vi "Discrete Lead Compensator Design.vi"() -> ()   [LabVIEW 2018]
uses:
  <vilib>/addons/Control Design/_Model Construction/Data Typedefs.llb/CD CtoD Conversion Method.ctl
  <vilib>/addons/Control Design/_Model Construction/Model Typedefs.llb/CD Transfer Function Model (MIMO).ctl
  <vilib>/addons/Control Design/_Model Construction/Model Typedefs.llb/CD General Elements.ctl
  <vilib>/addons/Control Design/_Model Construction/Model Typedefs.llb/CD Transfer Function Model (SISO).ctl
  <vilib>/addons/Control Design/_Utility/Rendering.llb/Rendering Transfer Function Options.ctl
  <vilib>/addons/Control Design/_Model Conversions/Continuous and Discrete.llb/Continuous and Discrete SubVI/cd_Convert Continuous to Discrete (TF).vi
  <vilib>/addons/Control Design/_Utility/Model Viewer.llb/Model Viewer SubVI/cd_Draw Transfer Function Equation (TF).vi
  <vilib>/addons/Control Design/_Model Construction/Model Creation.llb/Model Creation SubVI/cd_Create Transfer Function Model.vi
  <vilib>/addons/Control Design/_Model Interconnection/Model Interconnection.llb/Model Interconnection SubVI/cd_Matrix Multiply Models (TF and TF).vi
  <vilib>/addons/Control Design/_Dynamic Analysis/Dynamic Analysis.llb/Dynamic Analysis subVI/cd_Root Locus (Transfer Function).vi
  <vilib>/addons/Control Design/_Frequency Response Analysis/Frequency Response.llb/Frequency Response subVI/cd_Gain and Phase Margin (Transfer Function).vi
  <vilib>/addons/Control Design/_Model Interconnection/Model Interconnection.llb/Model Interconnection SubVI/cd_Unit Feedback (TF and TF).vi
  <vilib>/addons/Control Design/_Time Response Analysis/Time Response.llb/Time Response subVI/cd_Step Response (Transfer Function).vi
  <vilib>/addons/Control Design/_Utility/NI_CD_Model Viewer.lvlib
  <vilib>/addons/Control Design/_Model Construction/NI_LinSys_Model Typedefs.lvlib
  <vilib>/addons/Control Design/_Model Construction/NI_LinSys_Data Typedefs.lvlib
  <vilib>/addons/Control Design/_Utility/NI_LinSys_Rendering.lvlib
  <vilib>/addons/Control Design/_Model Conversions/NI_CD_Continuous and Discrete.lvlib
  <vilib>/addons/Control Design/_Dynamic Analysis/NI_CD_Dynamic Analysis.lvlib
  <vilib>/addons/Control Design/_Model Construction/NI_LinSys_Model Creation.lvlib
  <vilib>/addons/Control Design/_Model Interconnection/NI_CD_Model Interconnection.lvlib
  <vilib>/addons/Control Design/_Time Response Analysis/NI_CD_Time Response.lvlib
  <vilib>/addons/Control Design/_Frequency Response Analysis/NI_CD_Frequency Response.lvlib
panel:
  in  "stop":bool
  out "Damping":dbl=5.0
  in  "Overshoot (%)":dbl=5.0
  in  "Settling Time (s)":dbl=0.3
  in  "Tab Control":T1(tab)
  out "Magnitude Plot":cluster{"W":dbl[], "Magnitude":dbl[]}[](graph)
  out "Phase Plot":cluster{"W":dbl[], "Phase":dbl[]}[](graph)
  out "Root Locus Plot":cluster{"W":dbl[], "Magnitude":dbl[]}[](graph)
  out "Step Response":cluster{"W":dbl[], "Magnitude":dbl[]}[](graph)
  out "G_c(z)":picture
  in  "Pole":dbl=0.1 format="%#_13g"
  in  "Zero":dbl=0.1 format="%#_13g"
  in  "C":dbl=1.0 format="%#_13g"
  in  "K":dbl=1.0
  in  "tau":dbl=1.0 format="%#_13g"
  in  "Sampling period (s)":dbl=0.02 format="%#_13g"
  out "G_p(z)":picture
  # "Controls Board"
  # "Discrete Lead Compensator Design"
  # "Plant"
  # "Controller"
  # "Design Requirements"
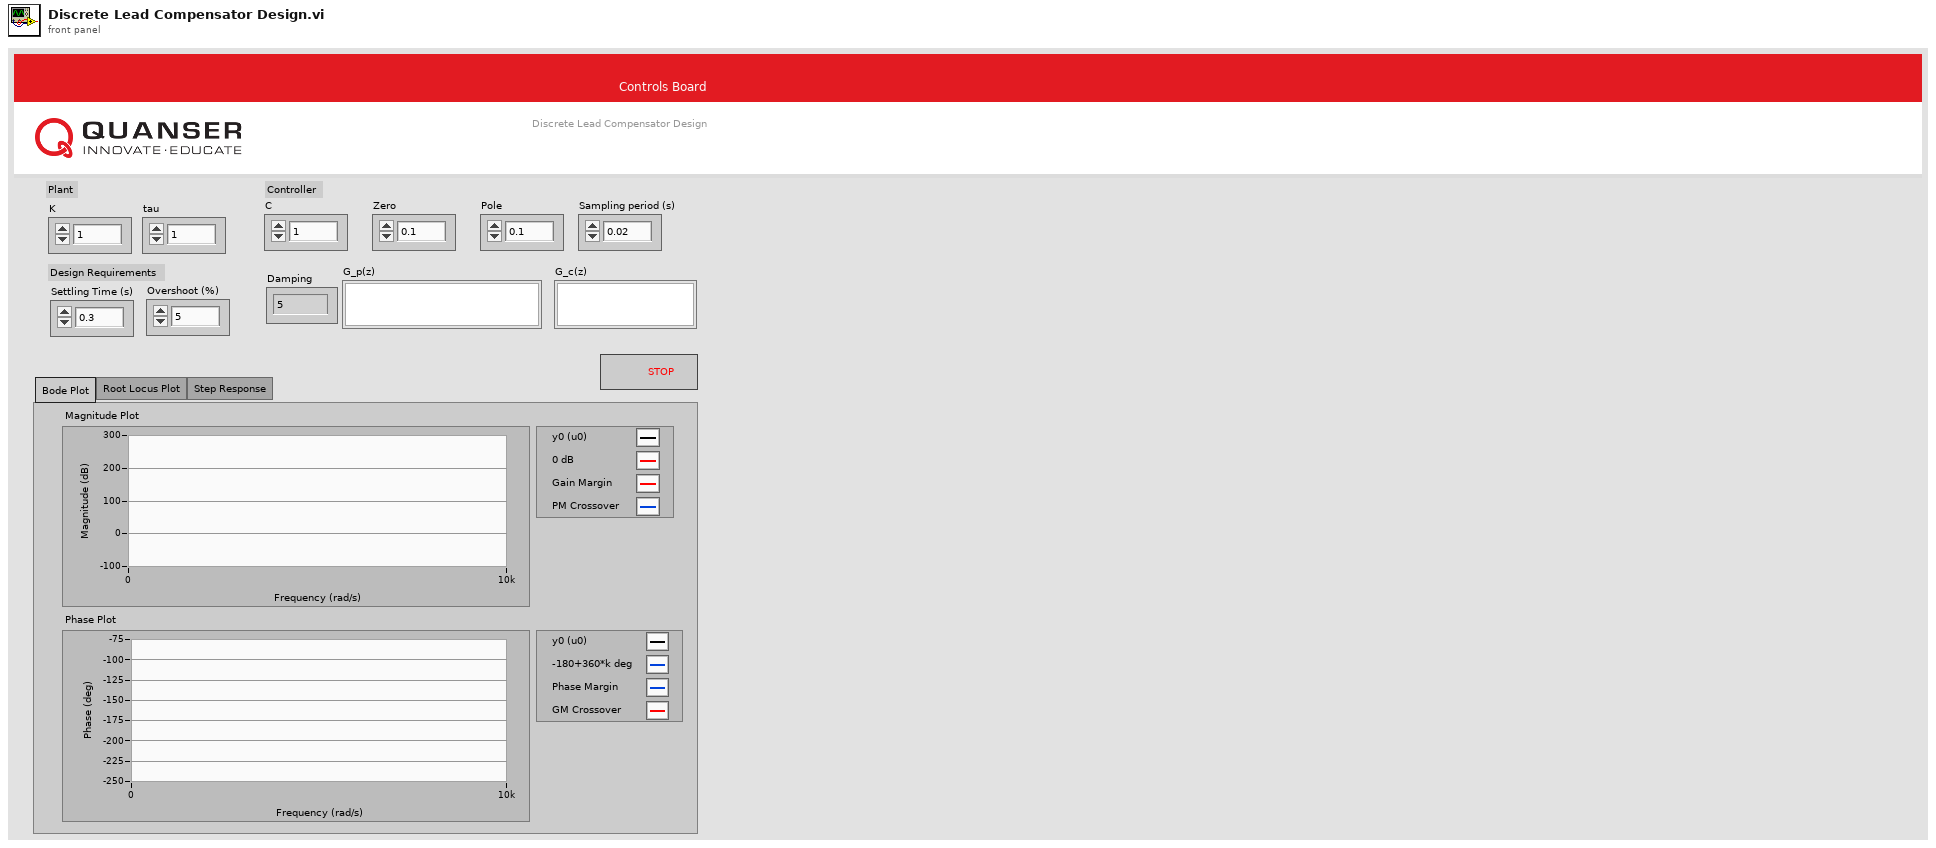
[diagram p1: front panel]
types:
  T1 = enum32{"Bode Plot", "Root Locus Plot", "Step Response"}
  T2 = typedef "NI_LinSys_Model Typedefs.lvlib/CD General Elements.ctl" = cluster{"Model name":string, "Input names":string[], "Output names":string[], "Input Delays":dbl[], "Output Delays":dbl[], "Sampling Time":dbl, "Notes":string}
  T3 = typedef "NI_LinSys_Rendering.lvlib/Rendering Transfer Function Options.ctl" = u16
  T4 = typedef "NI_LinSys_Model Typedefs.lvlib/CD Transfer Function Model (MIMO).ctl" = cluster{"properties":T2, "transfer function(s)":T5[][]}
  T5 = typedef "NI_LinSys_Model Typedefs.lvlib/CD Transfer Function Model (SISO).ctl" = cluster{"Numerator":dbl[], "Denominator":dbl[], "delay":dbl}
  T6 = typedef "NI_LinSys_Data Typedefs.lvlib/CD CtoD Conversion Method.ctl" = u16
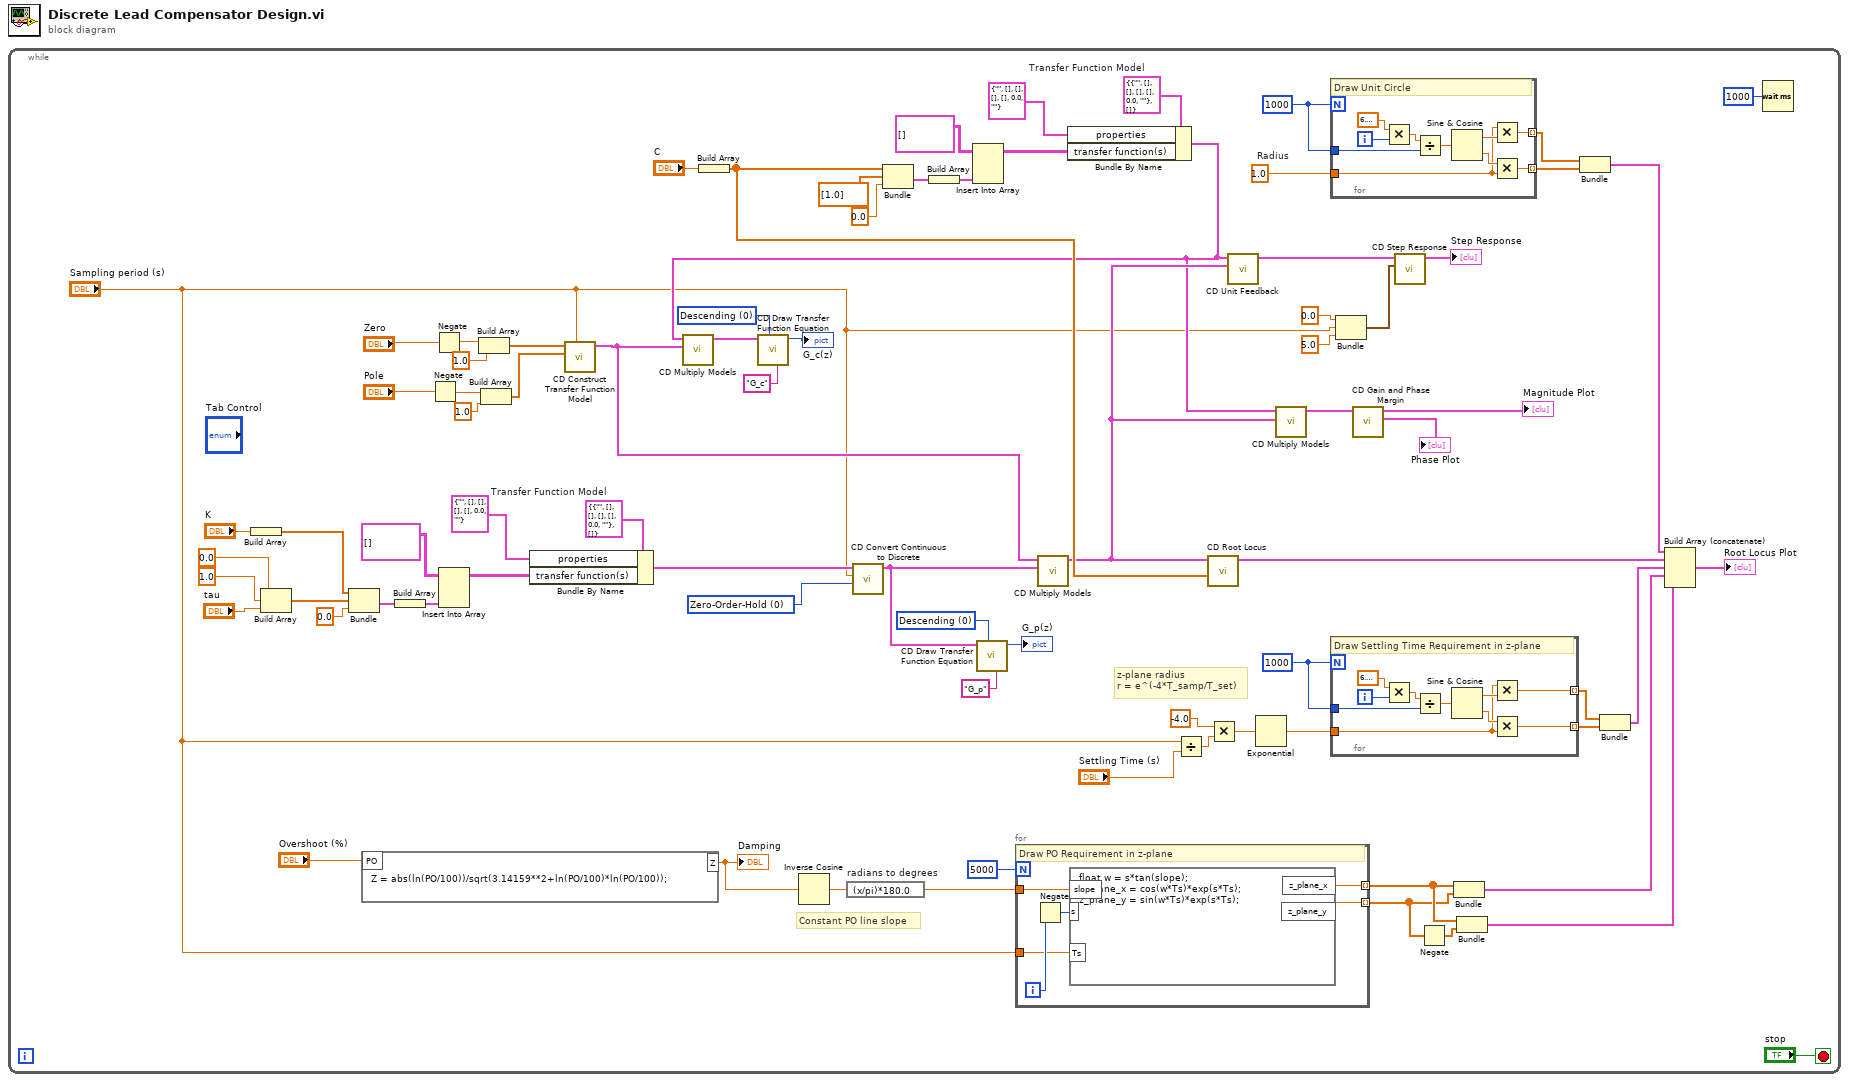
[diagram p0: block diagram]
diagram:
  n1 = while {
    stop <- "stop" stop-if-true
    w25 = 1000
    w31 = T3 0 items=["Descending", "Ascending", "Negative Power"] ("Display Format")
    w45 = T4 {"properties"={"Model name"="", "Input names"=[], "Output names"=[], "Input Delays"=[], "Output Delays"=[], "Sampling Time"=0.0, "Notes"=""}, "transfer function(s)"=[]}  # Transfer Function Model
    w55 = T4 {"properties"={"Model name"="", "Input names"=[], "Output names"=[], "Input Delays"=[], "Output Delays"=[], "Sampling Time"=0.0, "Notes"=""}, "transfer function(s)"=[]}  # Transfer Function Model
    w60 = T6 0 items=["Zero-Order-Hold", "Tustin (Bilinear)", "Prewarp", "Forward", "Backward", "Z-Transform", "First-Order-Hold", "Matched Pole-Zero"] ("Method")
    w57 = T3 0 items=["Descending", "Ascending", "Negative Power"] ("Display Format")
    w78 = 1.0  # Radius
    w81 = 1000
    # "Constant PO line slope"
    # "z-plane radius\nr = e^(-4*T_samp/T_set)"
    n2 = Build Array ("Build Array 5")("K") -> (w69:dbl[])
    n3 = Build Array ("Build Array 4")(0.0, 1.0, "tau") -> (w66:dbl[])
    n4 = Bundle ("Bundle 3")(w69, w66, 0.0) -> (w61:cluster{dbl[], dbl[], dbl})  [unwired: 1 in]
    n5 = formula code="Z = abs(ln(PO/100))/sqrt(3.14159**2+ln(PO/100)*ln(PO/100));"("PO"="Overshoot (%)") -> ("Z"=w12:dbl)
    "Damping" <- w12
    n6 = Build Array ("Build Array 3")(w61) -> (w67:cluster{dbl[], dbl[], dbl}[])
    n7 = Negate ("Negate 2")(x="Pole") -> (-x=w77:dbl)
    n8 = Negate(x="Zero") -> (-x=w76:dbl)
    n9 = Insert Into Array ("Insert Into Array 2")(array=cluster{dbl[], dbl[], dbl}[][] [], new element=w67) -> (w68:cluster{dbl[], dbl[], dbl}[][])  [unwired: 2 in]
    n10 = Build Array ("Build Array 7")(w76, 1.0 ("element")) -> (w73:dbl[])
    n11 = Build Array ("Build Array 8")(w77, 1.0 ("element")) -> (w75:dbl[])
    n12 = Bundle By Name(cluster=w55, "properties"=T2 {"Model name"="", "Input names"=[], "Output names"=[], "Input Delays"=[], "Output Delays"=[], "Sampling Time"=0.0, "Notes"=""}, "transfer function(s)"=w68) -> (w51:T4)
    n13 = call-poly <vilib>:"CD Construct Transfer Function Model.vi"("Sampling Time (s)"="Sampling period (s)", "Denominator"=w75, "Numerator"=w73) -> ("Transfer Function Model"=w28:T4)  [unwired: 7 in, 1 out]
    n14 = Build Array ("Build Array 6")("C") -> (w37:dbl[])
    n15 = Inverse Cosine(1:w12) -> (0:w11:dbl)
    n16 = expression code="(x/pi)*180.0" "radians to degrees"(w11) -> (w9:dbl)
    n17 = call-poly <vilib>:"CD Convert Continuous to Discrete.vi"("Method"=w60, "Sampling Time (s)"="Sampling period (s)", "Continuous Transfer Function Model"=w51) -> ("Discrete Transfer Function Model"=w50:T4)  [unwired: 7 in, 1 out]
    n18 = Bundle(w37, dbl[] [1.0], 0.0) -> (w40:cluster{dbl[], dbl[], dbl})  [unwired: 1 in]
    n19 = Build Array(w40) -> (w36:cluster{dbl[], dbl[], dbl}[])
    n20 = Insert Into Array(array=cluster{dbl[], dbl[], dbl}[][] [], new element=w36) -> (w39:cluster{dbl[], dbl[], dbl}[][])  [unwired: 2 in]
    n21 = call-poly <vilib>:"CD Draw Transfer Function Equation.vi"("Function Name (empty)"="G_p", "Display Format"=w57, "Transfer Function Model"=w50) -> ("Equation"=→"G_p(z)":picture)  [unwired: 6 in, 2 out]
    n22 = for {
      N: 5000 -> [_]
      tunnel: w9 -> [w85]
      tunnel: [w87] -> w6 mode=indexing
      tunnel: [w86] -> w4 mode=indexing
      tunnel: "Sampling period (s)" -> [w82]
      i -> [w84]
      # "Draw PO Requirement in z-plane"
      n23 = Negate(x=w84) -> (-x=w83:i32)
      n24 = formula code="float w = s*tan(slope);\nz_plane_x = cos(w*Ts)*exp(s*Ts);\nz_plane_y = sin(w*Ts)*exp(s*Ts);"("slope"=w85, "s"=w83, "Ts"=w82) -> ("z_plane_x"=w87:dbl, "z_plane_y"=w86:dbl)
    }
    n25 = call-poly <vilib>:"CD Multiply Models.vi"("Model 2"=w50, "Model 1"=w28) -> ("Model Out"=w14:T4)  [unwired: 8 in, 1 out]
    n26 = Bundle By Name(cluster=w45, "properties"=T2 {"Model name"="", "Input names"=[], "Output names"=[], "Input Delays"=[], "Output Delays"=[], "Sampling Time"=0.0, "Notes"=""}, "transfer function(s)"=w39) -> (w13:T4)
    n27 = call-poly <vilib>:"CD Multiply Models.vi"("Model 2"=w28, "Model 1"=w13) -> ("Model Out"=w29:T4)  [unwired: 8 in, 1 out]
    n28 = call-poly <vilib>:"CD Draw Transfer Function Equation.vi"("Function Name (empty)"="G_c", "Display Format"=w31, "Transfer Function Model"=w29) -> ("Equation"=→"G_c(z)":picture)  [unwired: 6 in, 2 out]
    n29 = Divide(x="Sampling period (s)", y="Settling Time (s)") -> (x/y=w18:dbl)
    n30 = call-poly <vilib>:"CD Root Locus.vi"("Gain"=w37, "Transfer Function Model"=w14) -> ("Root Locus Graph"=w70:cluster{dbl[], dbl[]}[])  [unwired: 6 in, 3 out]
    n31 = Multiply(x=-4.0, y=w18) -> (x*y=w20:dbl)
    n32 = call-poly <vilib>:"CD Unit Feedback.vi"("Model 2"=w14, "Model 1"=w13) -> ("Closed-Loop Model"=w46:T4)  [unwired: 8 in, 1 out]
    n33 = Exponential(1:w20) -> (0:w17:dbl)
    n34 = call-poly <vilib>:"CD Multiply Models.vi"("Model 2"=w14, "Model 1"=w13) -> ("Model Out"=w21:T4)  [unwired: 8 in, 1 out]
    n35 = for {
      N: w81 -> [_]
      tunnel: w81 -> [w105]
      tunnel: [w99] -> w80 mode=indexing
      tunnel: [w98] -> w79 mode=indexing
      tunnel: w78 -> [w100]
      i -> [w103]
      # "Draw Unit Circle"
      n36 = Multiply(x=6.283185307179586, y=w103) -> (x*y=w107:dbl)
      n37 = Divide(x=w107, y=w105) -> (x/y=w106:dbl)
      n38 = Sine & Cosine(0:w106) -> (1:w102:dbl, 2:w101:dbl)
      n39 = Multiply(x=w100, y=w102) -> (x*y=w99:dbl)
      n40 = Multiply(x=w101, y=w100) -> (x*y=w98:dbl)
    }
    n41 = for {
      N: w25 -> [_]
      tunnel: w25 -> [w95]
      tunnel: [w89] -> w26 mode=indexing
      tunnel: [w88] -> w27 mode=indexing
      tunnel: w17 -> [w90]
      i -> [w93]
      # "Draw Settling Time Requirement in z-plane"
      n42 = Multiply(x=6.283185307179586, y=w93) -> (x*y=w97:dbl)
      n43 = Divide(x=w97, y=w95) -> (x/y=w96:dbl)
      n44 = Sine & Cosine(0:w96) -> (1:w92:dbl, 2:w91:dbl)
      n45 = Multiply(x=w90, y=w92) -> (x*y=w89:dbl)
      n46 = Multiply(x=w91, y=w90) -> (x*y=w88:dbl)
    }
    n47 = Bundle(0.0, "Sampling period (s)"="Sampling period (s)", 5.0) -> (w47:cluster{dbl, "Sampling period (s)":dbl, dbl})  [unwired: 1 in]
    n48 = call-poly <vilib>:"CD Gain and Phase Margin.vi"("Transfer Function Model"=w21) -> ("Phase Plot"=→"Phase Plot":cluster{"W":dbl[], "Phase":dbl[]}[], "Magnitude Plot"=→"Magnitude Plot":cluster{"W":dbl[], "Magnitude":dbl[]}[])  [unwired: 6 in, 3 out]
    n49 = call-poly <vilib>:"CD Step Response.vi"("Time Range"=w47, "Transfer Function Model"=w46) -> ("Step Response Graph"=→"Step Response":cluster{"time":dbl[], dbl[]}[])  [unwired: 7 in, 2 out]
    n50 = Negate(x=w4) -> (-x=w5:dbl[])
    n51 = Bundle(w6, w4) -> (w7:cluster{dbl[], dbl[]})  [unwired: 1 in]
    n52 = Bundle(w6, w5) -> (w3:cluster{dbl[], dbl[]})  [unwired: 1 in]
    n53 = Bundle(w80, w79) -> (w53:cluster{dbl[], dbl[]})  [unwired: 1 in]
    n54 = Bundle(w26, w27) -> (w24:cluster{dbl[], dbl[]})  [unwired: 1 in]
    n55 = Build Array (concatenate)(w53, w70, w24, w7, w3) -> (→"Root Locus Plot":cluster{dbl[], dbl[]}[])
    n56 = Wait (ms)(milliseconds to wait=u32 1000) -> ()  [unwired: 1 out]
  }
